vi "AlliGator Set Phasor Reference.vi"(6 "Lifetime":dbl[unit], 7 "State Indicators Refnum":refnum<vi>, 8 "error in (no error)":errorcluster, 9 "Reference Number":i32, 10 "Plot Data Point":cluster{"X":dbl, "Y":dbl}, 11 "Phasor Graph Refnum":refnum<vi>) -> (0 "Error Out":errorcluster)   [LabVIEW 2021, in "AlliGator Phasor Ratio.lvlib"]
doc: "Updates phasor reference annotation in the Phasor Graph and sets corresponding status flag to True."
uses:
  AlliGator Phasor Ratio.lvlib
  GUI/AlliGator State Indicator.ctl
  Phasor Graph/AlliGator Phasor Graph.lvlib
  GUI/AlliGator GUI.lvlib
panel:
  # "see the AlliGator License on the block diagram (Ctrl+E or Window:Show Block Diagram)"
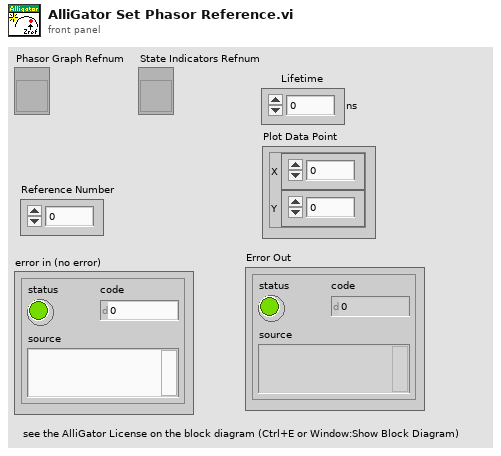
[diagram p1: front panel]
types:
  T1 = typedef "LVAnnotationListTypeDef.ctl" = cluster{"Name":string, "Color":u32, "Style":u8, "Point Style":u8, "Name Visible":bool, "Allow Drag":bool, "Annotation Mode":u32, "Plot":i32, "Index":i32, "Position":cluster{"X":dbl, "Y":dbl}, "X Scale":u32, "Y Scale":u32, "Show Arrow":bool, "Lock Name":bool, "Plot Area":i32, "Label Offset":cluster{"X":dbl, "Y":dbl}}[]
  T2 = cluster{"Name":string, "Color":u32, "Style":u8, "Point Style":u8, "Name Visible":bool, "Allow Drag":bool, "Annotation Mode":u32, "Plot":i32, "Index":i32, "Position":cluster{"X":dbl, "Y":dbl}, "X Scale":u32, "Y Scale":u32, "Show Arrow":bool, "Lock Name":bool, "Plot Area":i32, "Label Offset":cluster{"X":dbl, "Y":dbl}}
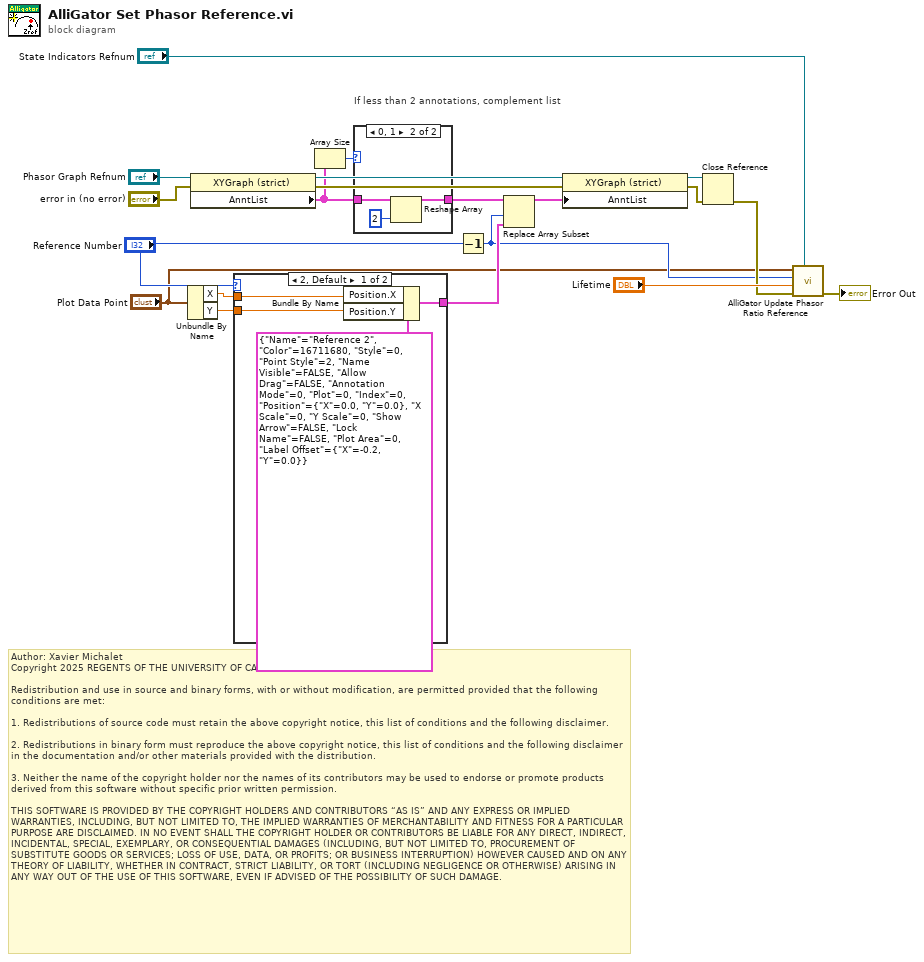
[diagram p0: block diagram]
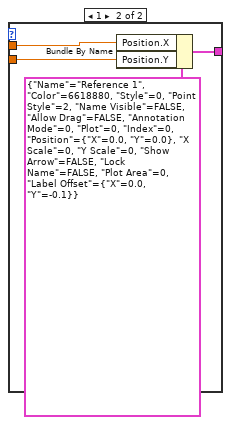
[diagram p3: hidden frame]
diagram:
  # "Author: Xavier Michalet\nCopyright 2025 REGENTS OF THE UNIVERSITY OF CALIFORNIA\n\nRedistribution and use in source and binary forms, with or without modification, are permitted provided that the following conditions are met:\n\n1. Redistributions of source code must retain the above copyright notice, this list of conditions and the following disclaimer.\n\n2. Redistributions in binary form must reproduce the above copyright notice, this list of conditions and the following disclaimer in the documentation and/or other materials provided with the distribution.\n\n3. Neither the name of the copyright holder nor the names of its contributors may be used to endorse or promote products derived from this software without specific prior written permission.\n\nTHIS SOFTWARE IS PROVIDED BY THE COPYRIGHT HOLDERS AND CONTRIBUTORS “AS IS” AND ANY EXPRESS OR IMPLIED WARRANTIES, INCLUDING, BUT NOT LIMITED TO, THE IMPLIED WARRANTIES OF MERCHANTABILITY AND FITNESS FOR A PARTICULAR PURPOSE ARE DISCLAIMED. IN NO EVENT SHALL THE COPYRIGHT HOLDER OR CONTRIBUTORS BE LIABLE FOR ANY DIRECT, INDIRECT, INCIDENTAL, SPECIAL, EXEMPLARY, OR CONSEQUENTIAL DAMAGES (INCLUDING, BUT NOT LIMITED TO, PROCUREMENT OF SUBSTITUTE GOODS OR SERVICES; LOSS OF USE, DATA, OR PROFITS; OR BUSINESS INTERRUPTION) HOWEVER CAUSED AND ON ANY THEORY OF LIABILITY, WHETHER IN CONTRACT, STRICT LIABILITY, OR TORT (INCLUDING NEGLIGENCE OR OTHERWISE) ARISING IN ANY WAY OUT OF THE USE OF THIS SOFTWARE, EVEN IF ADVISED OF THE POSSIBILITY OF SUCH DAMAGE."
  n1 = Unbundle By Name("Plot Data Point") -> ("X"=w13:dbl, "Y"=w12:dbl)
  n2 = property class="XYGraph (strict)"(reference="Phasor Graph Refnum", error in="error in (no error)") -> (reference out=w18:refnum<vi>, error out=w17:errorcluster, "AnntList"=w10:T1)
  n3 = case shown="2, Default" "Reference Number" {
    tunnel: w13 -> [w24 w27]
    tunnel: w12 -> [w23 w26]
    tunnel: [w22 w25] -> w14
    frame 2, Default {
      n4 = Bundle By Name(cluster=T2 {"Name"="Reference 2", "Color"=16711680, "Style"=0, "Point Style"=2, "Name Visible"=FALSE, "Allow Drag"=FALSE, "Annotation Mode"=0, "Plot"=0, "Index"=0, "Position"={"X"=0.0, "Y"=0.0}, "X Scale"=0, "Y Scale"=0, "Show Arrow"=FALSE, "Lock Name"=FALSE, "Plot Area"=0, "Label Offset"={"X"=-0.2, "Y"=0.0}} ("Cluster"), "Position.X"=w24, "Position.Y"=w23) -> (w22:T2)
    }
    frame 1 {
      n5 = Bundle By Name(cluster=T2 {"Name"="Reference 1", "Color"=6618880, "Style"=0, "Point Style"=2, "Name Visible"=FALSE, "Allow Drag"=FALSE, "Annotation Mode"=0, "Plot"=0, "Index"=0, "Position"={"X"=0.0, "Y"=0.0}, "X Scale"=0, "Y Scale"=0, "Show Arrow"=FALSE, "Lock Name"=FALSE, "Plot Area"=0, "Label Offset"={"X"=0.0, "Y"=-0.1}} ("Cluster"), "Position.X"=w27, "Position.Y"=w26) -> (w25:T2)
    }
  }
  n6 = Array Size(array=w10) -> (size(s)=w11:i32)
  n7 = case "If less than 2 annotations, complement list" shown="0, 1" w11 {
    tunnel: w10 -> [w29 w32]
    tunnel: [w29 w30] -> w9
    frame 2.., Default {
    }
    frame 0, 1 {
      n8 = Reshape Array(w32, 2 ("dimension size")) -> (w30:T1)
    }
  }
  n9 = Decrement(x="Reference Number") -> (x-1=w3:i32)
  n10 = Replace Array Subset(array=w9, new element=w14, index=w3) -> (w16:T1)
  n11 = property class="XYGraph (strict)"(reference=w18, error in=w17, "AnntList"=w16) -> (reference out=w15:refnum<vi>, error out=w8:errorcluster)
  n12 = Close Reference(reference=w15, error in (no error)=w8) -> (error out=w4:errorcluster)
  n13 = call "AlliGator Update Phasor Ratio Reference.vi"("State Indicators Refnum"="State Indicators Refnum", "error in (no error)"=w4, "Lifetime"="Lifetime", "Reference Idx (0 or 1)"=w3, "Phasor"="Plot Data Point") -> ("error out"=→"Error Out":errorcluster)  [unwired: 6 in]
